vi "StaticBrake Setter.vi"(0 "DeviceReference":T1, 3 "Update Frequency (Hz)":dbl=100.0) -> (4 "DeviceReference Out":T1)   [LabVIEW 2020]
doc: "Applies full neutral-brake by shorting motor leads together."
uses:
  DeviceReference.ctl
  <userlib>/CTRE_PhoenixTools/CTRE_PhoenixTools.lvlib
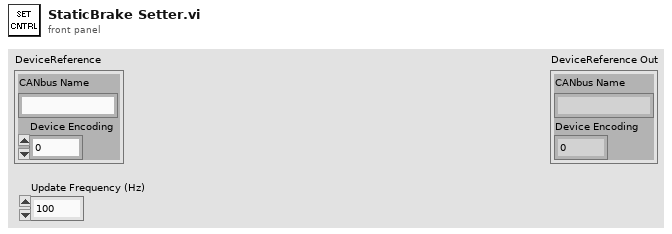
[diagram p1: front panel]
types:
  T1 = typedef "DeviceReference.ctl" = cluster{"CANbus Name":string, "Device Encoding":u32}
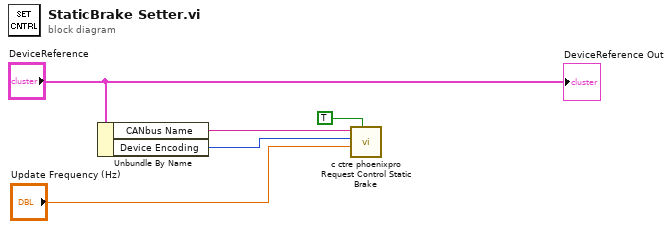
[diagram p0: block diagram]
diagram:
  n1 = Unbundle By Name("DeviceReference") -> ("CANbus Name"=w4:string, "Device Encoding"=w3:u32)
  n2 = call <userlib>:"c ctre phoenixpro Request Control Static Brake.vi"("cancelOtherRequests"=TRUE, "updateTime"="Update Frequency (Hz)", "ecuEncoding"=w3, "canbus"=w4) -> ()  [unwired: 6 in, 2 out]
  "DeviceReference Out" <- "DeviceReference"
